vi "XY Plot Buffer.vi"(9 "History Length":i32, 10 "Input 2":sgl, 11 "Input 1":sgl) -> (2 "Y Buffer":sgl[](array[numeric]), 3 "X Buffer":sgl[](array[numeric]))   [LabVIEW 2015, in "ECS-Host.lvlib"]
uses:
  ECS-Host.lvlib
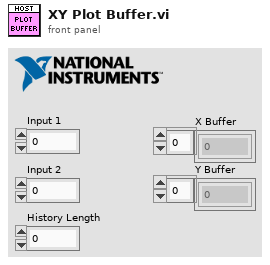
[diagram p1: front panel]
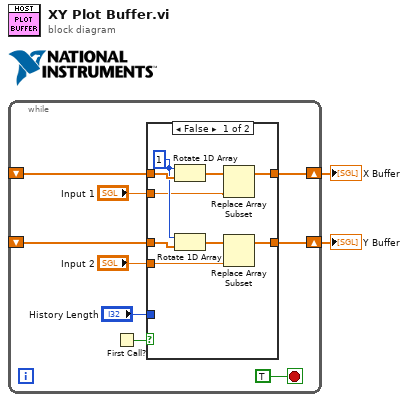
[diagram p0: block diagram]
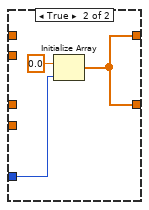
[diagram p2: hidden frame]
diagram:
  n1 = while {
    shift-right: [w9] -> w2
    shift-left: _ -> [w6]
    shift-right: [w8] -> w1
    shift-left: _ -> [w5]
    stop <- TRUE stop-if-true
    n2 = First Call?() -> (First Call?: T/F=w10:bool)
    n3 = case shown="False" w10 {
      tunnel: [w20 w23] -> w9
      tunnel: [w19 w23] -> w8
      tunnel: "History Length" -> [_ w21]
      tunnel: w6 -> [w18 _]
      tunnel: w5 -> [w16 _]
      tunnel: "Input 2" -> [w13 _]
      tunnel: "Input 1" -> [w12 _]
      frame False {
        w14 = 1 ("n")
        n4 = Rotate 1D Array(1:w18, 2:w14) -> (0:w17:sgl[])
        n5 = Rotate 1D Array(1:w16, 2:w14) -> (0:w15:sgl[])
        n6 = Replace Array Subset(array=w17, new element=w12) -> (w20:sgl[])  [unwired: 1 in]
        n7 = Replace Array Subset(array=w15, new element=w13) -> (w19:sgl[])  [unwired: 1 in]
      }
      frame True {
        n8 = Initialize Array(sgl 0.0 ("element"), w21) -> (w23:sgl[])
      }
    }
  }
  "X Buffer" <- w2
  "Y Buffer" <- w1
